vi "test Verify Class Roster.vi"(8 "error in":errorcluster, 11 "Test Case In":refnum<class "LUnit Extensions Tests.lvclass">) -> (0 "error out":errorcluster, 3 "Test Case Out":refnum<class "LUnit Extensions Tests.lvclass">)   [LabVIEW 2020, in "LUnit Extensions Tests.lvclass"]
uses:
  LUnit Extensions Tests.lvclass
  C:/Program Files/National Instruments/LabVIEW 2026/vi.lib/Astemes/LUnit/Test Case.lvclass
  Source/Approval Tests/Options/Options.lvclass/Options.ctl
  Source/Approval Tests/Naming Data/Naming Data.lvclass/Naming Data.ctl
  <vilib>/Astemes/LUnit/Test Case.lvclass/Test Case.ctl
  0af6d9d6-a82c-41a4-957f-9537b381c366.vi
  0af6d9d6-a82c-41a4-957f-9537b381c366.vi/1e051690-6811-4db0-8b8f-f6ad9423d026.vi
  Source/Approval Tests/Replace if Empty.vi
  <vilib>/Astemes/LUnit/Palette/Pass If.vi
  Source/Approval Tests/Options/Update Test Name if Not Defined.vi
  Source/Approval Tests/Verify Core.vi
  0af6d9d6-a82c-41a4-957f-9537b381c366.vi/1e051690-6811-4db0-8b8f-f6ad9423d026.vi/93c5622b-9fb7-41e0-8c76-3fde37e94e34.vi
  Source/Approval Tests/Options/Read Scrubber.vi
  <vilib>/Astemes/LUnit/Core/LUnit Test Case/Private/Append Fail Result.vi
  <vilib>/Astemes/LUnit/Core/LUnit Test Case/Private/Append Pass Result.vi
  Source/Approval Tests/Naming Data/Read Test VI Name.vi
  Source/Approval Tests/Naming Data/Write Test VI Name.vi
  Source/Approval Tests/Options/Read Namer.vi
  Source/Approval Tests/Options/Read Naming Data.vi
  Source/Approval Tests/Options/Read Reporter.vi
  Source/Approval Tests/Options/Read Text Comparator.vi
  0af6d9d6-a82c-41a4-957f-9537b381c366.vi/1e051690-6811-4db0-8b8f-f6ad9423d026.vi/93c5622b-9fb7-41e0-8c76-3fde37e94e34.vi/04cb982b-2eda-40d0-8d7e-90f8e0b569b2.vi
  <vilib>/Astemes/LUnit/Core/LUnit Test Case/Private/Run In UI.vi
  0af6d9d6-a82c-41a4-957f-9537b381c366.vi/1e051690-6811-4db0-8b8f-f6ad9423d026.vi/93c5622b-9fb7-41e0-8c76-3fde37e94e34.vi/04cb982b-2eda-40d0-8d7e-90f8e0b569b2.vi/04ec6d97-7b7c-4123-b264-4b7eb8a41208.vi
  <vilib>/Utility/error.llb/Clear Errors.vi
  <vilib>/PNR/JSONtext Object Serialization/Generic Object Serializer/Generic Object Serializer.lvclass
  C:/Program Files/National Instruments/LabVIEW 2026/vi.lib/JDP Science/JSONtext/LVClass Serializer/JSONtext LVClass Serializer.lvclass
  Source/Approval Tests/Options/Add Label to Namer.vi
  <vilib>/JDP Science/JSONtext/Variant to JSON Text.vi
  Source/Approval Tests/conv EOL.vi
  <vilib>/Utility/libraryn.llb/Check if File or Folder Exists.vi
  Source/Approval Tests/Reporter/Report.vi
  Source/Approval Tests/Scrubber/Scrubber.lvclass
  Source/Approval Tests/Namer/Namer.lvclass
  Source/Approval Tests/Naming Data/Naming Data.lvclass
  Source/Approval Tests/Reporter/Reporter.lvclass
  Source/Approval Tests/Text Comparator/Text Comparator.lvclass
  Source/Approval Tests/Options/Options.lvclass
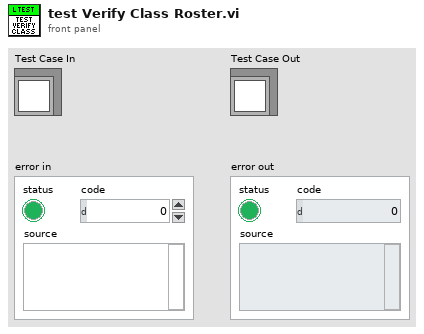
[diagram p1: front panel]
types:
  T1 = cluster{"Subject":string, "Teacher":cluster{"First Name":string, "Last Name":string}, "Assignments":cluster{"Description":string, "Grades":map{cluster{"First Name":string, "Last Name":string}, i32}}[], "Roster":cluster{"First Name":string, "Last Name":string}[]}
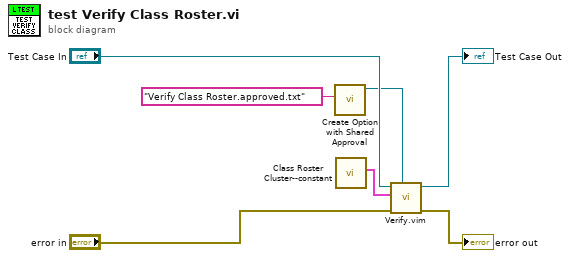
[diagram p0: block diagram]
diagram:
  n1 = call "Create Option with Shared Approval.vi"("Filename"="Verify Class Roster.approved.txt") -> ("Options outs"=w1:refnum<class "Options.lvclass">)  [unwired: 10 in]
  n2 = call "Class Roster Cluster--constant.vi"() -> ("Class Roster"=w3:T1)  [unwired: 11 in]
  n3 = call "Verify.vim"("Options"=w1, "error in"="error in", "Test Data"=w3, "LUnit Test Case In"="Test Case In") -> ("error out"=→"error out":errorcluster, "LUnit Test Case Out"=→"Test Case Out":refnum<class "LUnit Extensions Tests.lvclass">)  [unwired: 6 in]
